vi "updateBfieldSingle.vi"(7 "deadband":dbl, 8 "error in (no error)":errorcluster, 9 "B [T] in":dbl, 10 "Force upodate (F)":bool, 11 "MagSpecCamera in":refnum<class "MagSpecCamera.lvclass">) -> (0 "error out":errorcluster, 3 "MagSpecCamera out":refnum<class "MagSpecCamera.lvclass">)   [LabVIEW 2020, in "MagSpecCamera.lvclass"]
uses:
  MagSpecCamera.lvclass
  MagSpecCamera.lvclass/MagSpecCamera.ctl
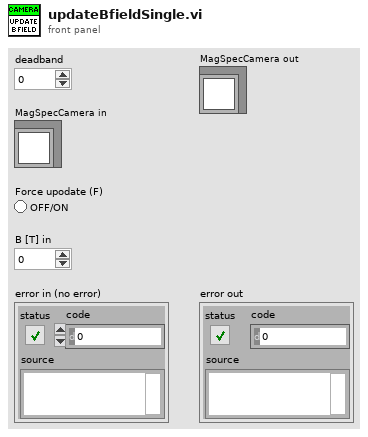
[diagram p1: front panel]
types:
  T1 = typedef "OnOffTypeDef.ctl" = enum16{"off", "on"}
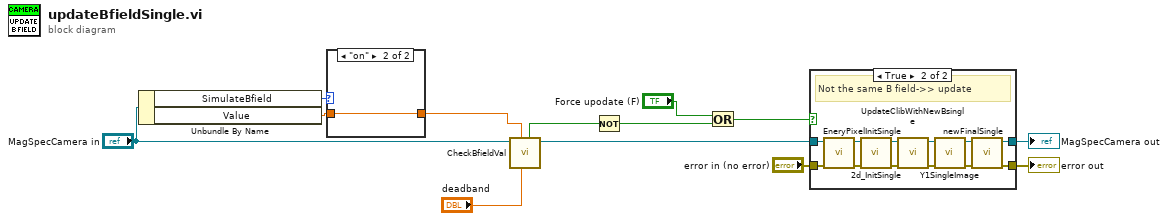
[diagram p0: block diagram]
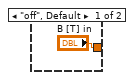
[diagram p2: hidden frame]
diagram:
  n1 = Unbundle By Name("MagSpecCamera in") -> ("SimulateBfield"=w3:T1, "Value"=w1:dbl)
  n2 = case shown="\"on\"" w3 {
    tunnel: ["B [T] in" w15] -> w2
    tunnel: w1 -> [_ w15]
    frame "off", Default {
    }
    frame "on" {
    }
  }
  n3 = call "CheckBfieldVal .vi"("deadband"="deadband", "B [T] new"=w2, "MagSpecCamera in"="MagSpecCamera in") -> ("MagSpecCamera in"=w7:refnum<class "MagSpecCamera.lvclass">, "Same?"=w12:bool)  [unwired: 7 in]
  n4 = Not(x=w12) -> (.not. x?=w11:bool)
  n5 = Or(x="Force upodate (F)", y=w11) -> (x .or. y?=w9:bool)
  n6 = case shown="True" w9 {
    tunnel: [w16 w28] -> w6
    tunnel: [w17 w24] -> w5
    tunnel: "error in (no error)" -> [w17 w18]
    tunnel: w7 -> [w16 w22]
    frame False {
    }
    frame True {
      # "Not the same B field->> update"
      n7 = call "EneryPixelInitSingle.vi"("error in (no error)"=w18, "MagSpecCamera in"=w22) -> ("error out"=w23:errorcluster, "MagSpecCamera in"=w21:refnum<class "MagSpecCamera.lvclass">)  [unwired: 8 in]
      n8 = call "2d_InitSingle.vi"("error in (no error)"=w23, "MagSpecCamera in"=w21) -> ("error out"=w19:errorcluster, "MagSpecCamera in"=w20:refnum<class "MagSpecCamera.lvclass">)  [unwired: 8 in]
      n9 = call "UpdateClibWithNewBsingle.vi"("error in (no error)"=w19, "MagSpecCamera in"=w20) -> ("error out"=w26:errorcluster, "MagSpecCamera in"=w27:refnum<class "MagSpecCamera.lvclass">)  [unwired: 8 in]
      n10 = call "Y1SingleImage.vi"("error in (no error)"=w26, "MagSpecCamera in"=w27) -> ("error out"=w25:errorcluster, "MagSpecCamera in"=w29:refnum<class "MagSpecCamera.lvclass">)  [unwired: 8 in]
      n11 = call "newFinalSingle.vi"("error in (no error)"=w25, "MagSpecCamera in"=w29) -> ("error out"=w24:errorcluster, "MagSpecCamera in"=w28:refnum<class "MagSpecCamera.lvclass">)  [unwired: 8 in]
    }
  }
  "MagSpecCamera out" <- w6
  "error out" <- w5
